vi "_CSTK_Button_Icon_Config_PreviewImage.vi"(7 "State in":T1) -> (3 "Preview Image":picture caption="预览图片")   [LabVIEW 2015, in "CSTK_Button_Icon.xctl"]
uses:
  CSTK_Button_Icon.xctl
  CSTK_Button_Icon_Status.ctl
  TypeDefinitions/_CSTK_Button_Icon_ButtonSize.ctl
  <vilib>/Utility/miscctls.llb/LVBoundsTypeDef.ctl
  TypeDefinitions/_CSTK_Button_Icon_LogoImage.ctl
  <vilib>/picture/picture.llb/imagedata.ctl
  TypeDefinitions/_CSTK_Button_Icon_LogoProperties.ctl
  TypeDefinitions/_CSTK_Button_Icon_LogoProperties_Data.ctl
  TypeDefinitions/_CSTK_Button_Icon_TextString.ctl
  TypeDefinitions/_CSTK_Button_Icon_TextProperties.ctl
  TypeDefinitions/_CSTK_Button_Icon_TextProperties_Data.ctl
  TypeDefinitions/_CSTK_Button_Icon_TextProperties_FontStyle.ctl
  TypeDefinitions/_CSTK_Button_Icon_BGColor.ctl
  TypeDefinitions/_CSTK_Button_Icon_BorderColor.ctl
  TypeDefinitions/_CSTK_Button_Icon_BorderProperties.ctl
  TypeDefinitions/_CSTK_Button_Icon_BorderProperties_Data.ctl
  TypeDefinitions/_CSTK_Button_Icon_CurrentBGImage.ctl
  TypeDefinitions/_CSTK_Button_Icon_DrawAreaSize.ctl
  TypeDefinitions/_CSTK_Button_Icon_TextStartOffset.ctl
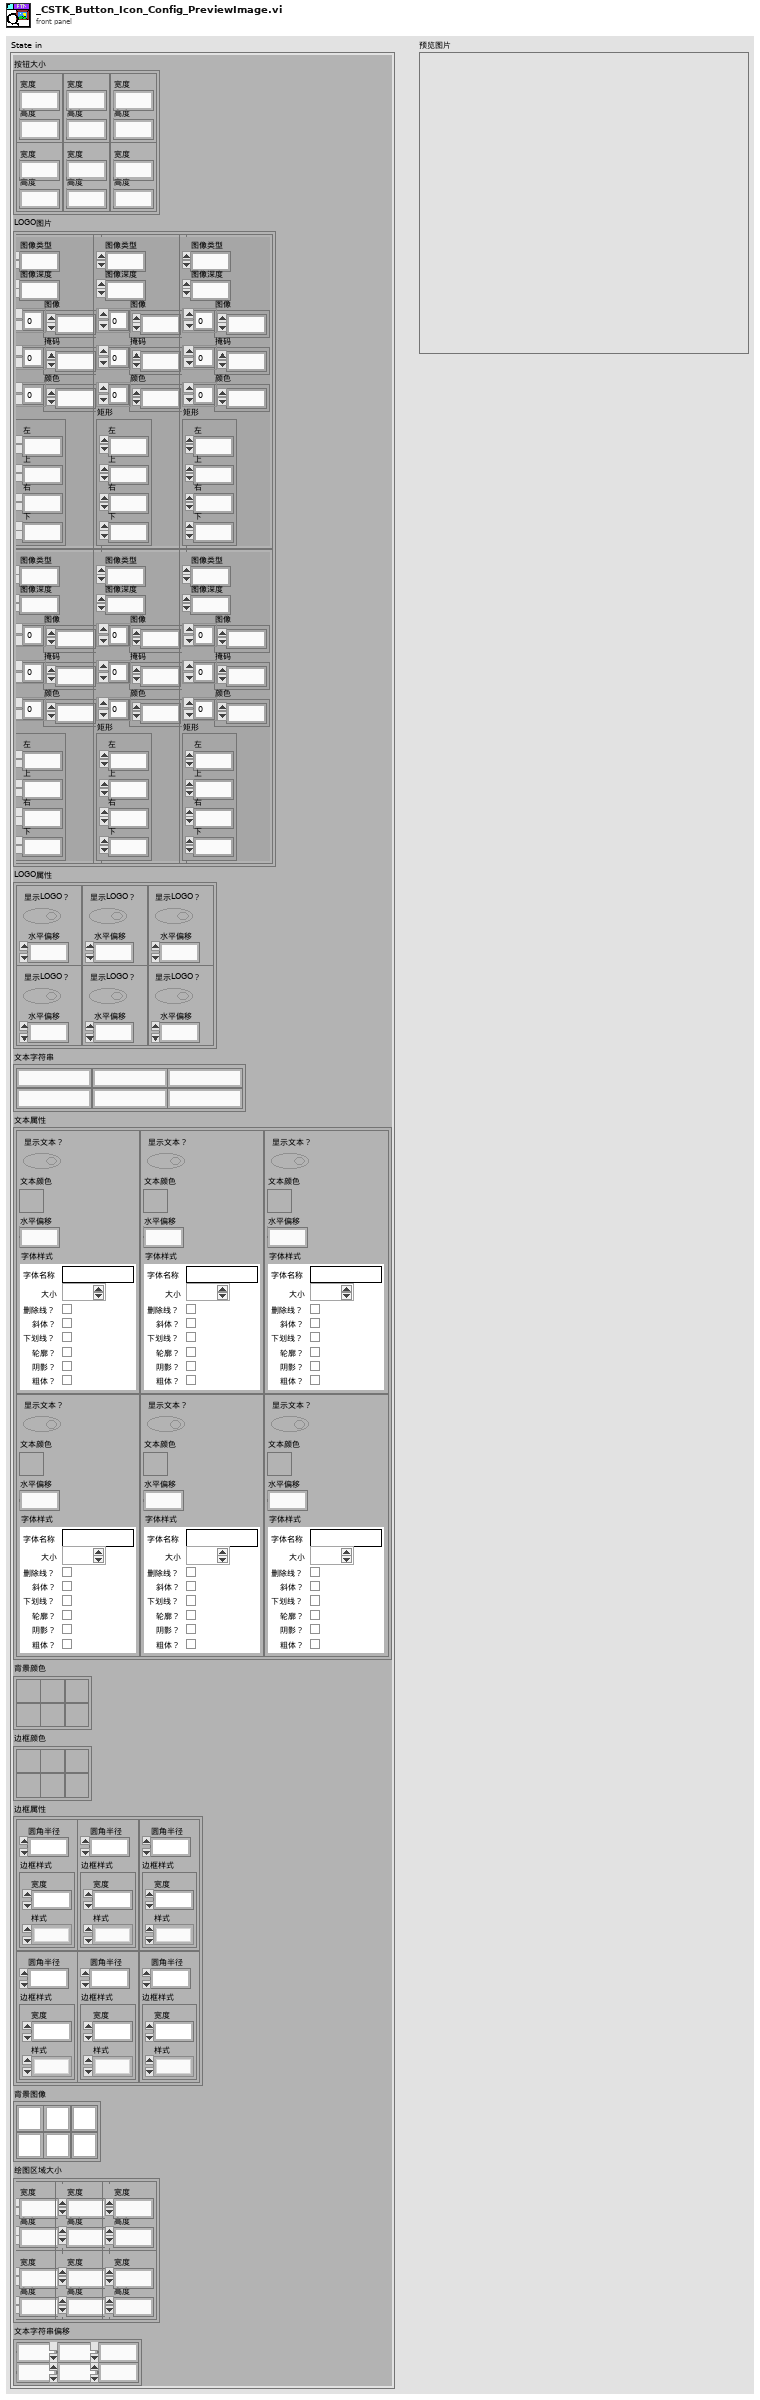
[diagram p1: front panel]
types:
  T1 = typedef "CSTK_Button_Icon.xctl/CSTK_Button_Icon_Status.ctl" = cluster{"ButtonSize":T2, "Logo Image":T4, "Logo Properties":T6, "Text String":T8, "Text Properties":T9, "BG Color":T12, "Border Color":T13, "Border Properties":T14, "Current BG Image":T16, "DrawAreaSize":T17, "Text String Offset":T18}
  T2 = typedef "CSTK_Button_Icon.xctl/_CSTK_Button_Icon_ButtonSize.ctl" = cluster{"False":T3, "True":T3, "True to False":T3, "False to True":T3, "Hover in False":T3, "Hover in True":T3}
  T3 = typedef "LVBoundsTypeDef.ctl" = cluster{"Width":u32, "Height":u32}
  T4 = typedef "CSTK_Button_Icon.xctl/_CSTK_Button_Icon_LogoImage.ctl" = cluster{"False":T5, "True":T5, "True to False":T5, "False to True":T5, "Hover in False":T5, "Hover in True":T5}
  T5 = typedef "imagedata.ctl" = cluster{"image type":i32, "image depth":i32, "image":u8[], "mask":u8[], "colors":u32[], "Rectangle":cluster{"left":i16, "top":i16, "right":i16, "bottom":i16}}
  T6 = typedef "CSTK_Button_Icon.xctl/_CSTK_Button_Icon_LogoProperties.ctl" = cluster{"False":T7, "True":T7, "True to False":T7, "False to True":T7, "Hover in False":T7, "Hover in True":T7}
  T7 = typedef "CSTK_Button_Icon.xctl/_CSTK_Button_Icon_LogoProperties_Data.ctl" = cluster{"Display Logo?":bool, "Horizontal Offset":i16}
  T8 = typedef "CSTK_Button_Icon.xctl/_CSTK_Button_Icon_TextString.ctl" = cluster{"False":string, "True":string, "True to False":string, "False to True":string, "Hover in False":string, "Hover in True":string}
  T9 = typedef "CSTK_Button_Icon.xctl/_CSTK_Button_Icon_TextProperties.ctl" = cluster{"False":T10, "True":T10, "True to False":T10, "False to True":T10, "Hover in False":T10, "Hover in True":T10}
  T10 = typedef "CSTK_Button_Icon.xctl/_CSTK_Button_Icon_TextProperties_Data.ctl" = cluster{"Display Text?":bool, "Text Color":u32, "Horizontal Offset":i16, "Font Style":T11}
  T11 = typedef "CSTK_Button_Icon.xctl/_CSTK_Button_Icon_TextProperties_FontStyle.ctl" = cluster{"Font Name":string, "Size":i16, "Strikeout?":bool, "Italic?":bool, "Underline?":bool, "Outline?":bool, "Shadow?":bool, "Bold?":bool}
  T12 = typedef "CSTK_Button_Icon.xctl/_CSTK_Button_Icon_BGColor.ctl" = cluster{"False":u32, "True":u32, "True to False":u32, "False to True":u32, "Hover in False":u32, "Hover in True":u32}
  T13 = typedef "CSTK_Button_Icon.xctl/_CSTK_Button_Icon_BorderColor.ctl" = cluster{"False":u32, "True":u32, "True to False":u32, "False to True":u32, "Hover in False":u32, "Hover in True":u32}
  T14 = typedef "CSTK_Button_Icon.xctl/_CSTK_Button_Icon_BorderProperties.ctl" = cluster{"False":T15, "True":T15, "True to False":T15, "False to True":T15, "Hover in False":T15, "Hover in True":T15}
  T15 = typedef "CSTK_Button_Icon.xctl/_CSTK_Button_Icon_BorderProperties_Data.ctl" = cluster{"Radius":i16, "Border Style":cluster{"Width":u16, "Style":enum32{"Solid", "Dash", "Dot", "DashDot", "DashDotDot"}}}
  T16 = typedef "CSTK_Button_Icon.xctl/_CSTK_Button_Icon_CurrentBGImage.ctl" = cluster{"False":picture, "True":picture, "True to False":picture, "False to True":picture, "Hover in False":picture, "Hover in True":picture}
  T17 = typedef "CSTK_Button_Icon.xctl/_CSTK_Button_Icon_DrawAreaSize.ctl" = cluster{"False":T3, "True":T3, "True to False":T3, "False to True":T3, "Hover in False":T3, "Hover in True":T3}
  T18 = typedef "CSTK_Button_Icon.xctl/_CSTK_Button_Icon_TextStartOffset.ctl" = cluster{"False":i32, "True":i32, "True to False":i32, "False to True":i32, "Hover in False":i32, "Hover in True":i32}
  T19 = cluster{"left":i16, "top":i16, "right":i16, "bottom":i16}
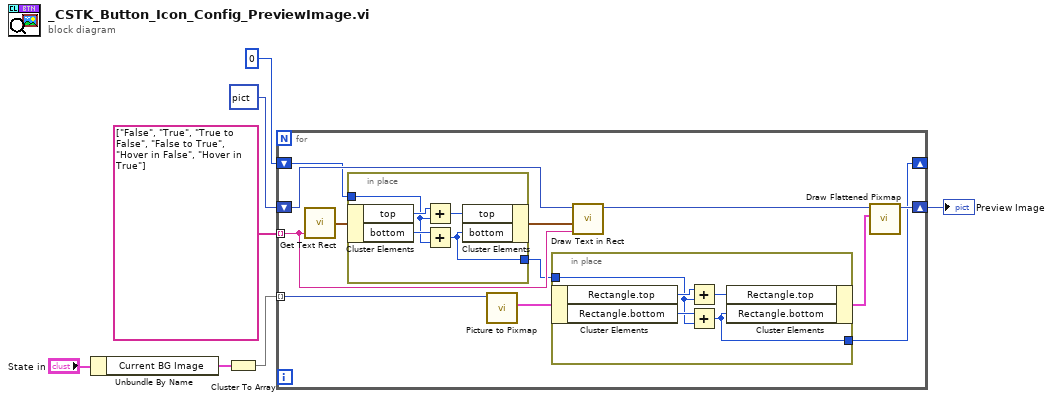
[diagram p0: block diagram]
diagram:
  n1 = Unbundle By Name("State in") -> ("Current BG Image"=w7:T16)
  n2 = Cluster To Array(cluster=w7) -> (array=w6:picture[])
  n3 = for {
    tunnel: w6 -> [w19] mode=indexing
    shift-right: [w17] -> w3
    shift-left: picture data[5B] ("Current BG Image.True") -> [w14]
    shift-right: [w15] -> _
    shift-left: i16 0 ("y") -> [w9]
    tunnel: string[] ["False", "True", "True to False", "False to True", "Hover in False", "Hover in True"] ("数组") -> [w12] mode=indexing
    n4 = call <vilib>:"Get Text Rect.vi"("text"=w12) -> ("rect"=w11:T19)  [unwired: 8 in]
    n5 = in-place {
      in-place-border: w9 -> [w21]
      in-place-border: [w20] -> w8
      n6 = in-place-cluster #1(w11) -> ("top"=w24:i16, "bottom"=w22:i16)
      n7 = Add(x=w24, y=w21) -> (x+y=w23:i16)
      n8 = Add(x=w22, y=w21) -> (x+y=w20:i16)
      n9 = in-place-cluster #1("top"=w23, "bottom"=w20) -> (w10:T19)
    }
    n10 = call <vilib>:"Picture to Pixmap.vi"("picture"=w19) -> ("image data"=w18:T5)  [unwired: 9 in, 1 out]
    n11 = in-place {
      in-place-border: w8 -> [w26]
      in-place-border: [w25] -> w15
      n12 = in-place-cluster #2(w18) -> ("Rectangle.top"=w29:i16, "Rectangle.bottom"=w27:i16)
      n13 = Add(x=w29, y=w26) -> (x+y=w28:i16)
      n14 = Add(x=w27, y=w26) -> (x+y=w25:i16)
      n15 = in-place-cluster #2("Rectangle.top"=w28, "Rectangle.bottom"=w25) -> (w16:T5)
    }
    n16 = call <vilib>:"Draw Text in Rect.vi"("text"=w12, "rect"=w10, "picture"=w14) -> ("new picture"=w13:picture)  [unwired: 8 in]
    n17 = call <vilib>:"Draw Flattened Pixmap.vi"("image data"=w16, "picture"=w13) -> ("new picture"=w17:picture)  [unwired: 7 in]
  }
  "Preview Image" <- w3
